vi "SP Determine Active Plot.vi"(0 "CH Index":i32, 1 "Trace Orientation":enum32{"Overlay", "Split"}(radio), 2 "Plot Orientation":enum32{"Single", "Dual", "Quad"}(radio), 3 "Plots Tab Control":refnum<vi>) -> ()   [LabVIEW 2011]
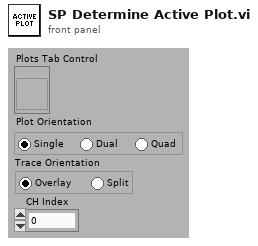
[diagram p1: front panel]
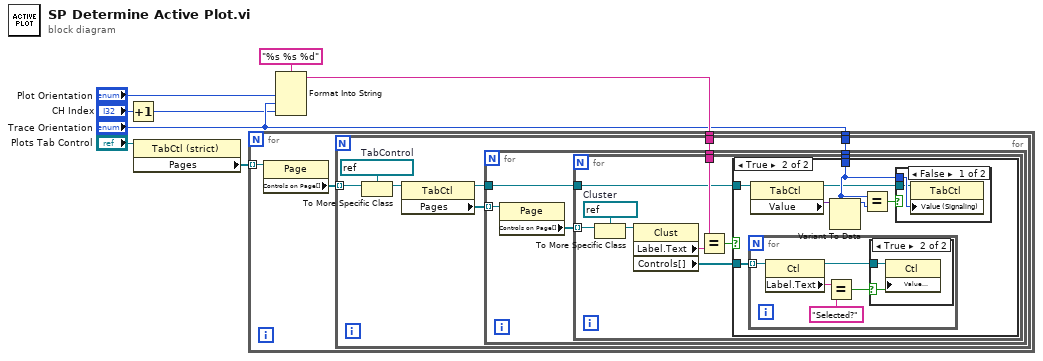
[diagram p0: block diagram]
diagram:
  n1 = Increment(x="CH Index") -> (x+1=w1:i32)
  n2 = property class="TabCtl (strict)"(reference="Plots Tab Control") -> ("Pages"=w4:refnum<vi>[])  [unwired: 1 in, 2 out]
  n3 = Format Into String(format string="%s %s %d", "Plot Orientation", "Trace Orientation", w1) -> (resulting string=w3:string)  [unwired: 2 in, 1 out]
  n4 = for {
    tunnel: w4 -> [w12] mode=indexing
    tunnel: w3 -> [w10]
    tunnel: "Trace Orientation" -> [w9]
    n5 = property class="Page"(reference=w12) -> ("Controls on Page[]"=w11:refnum<vi>[])  [unwired: 1 in, 2 out]
    n6 = for {
      tunnel: w11 -> [w19] mode=indexing
      tunnel: w10 -> [w15]
      tunnel: w9 -> [w13]
      w18 = refnum<vi> refnum  # TabControl
      n7 = To More Specific Class(target class=w18, reference=w19) -> (specific class reference=w17:refnum<vi>)  [unwired: 1 in, 1 out]
      n8 = property class="TabCtl"(reference=w17) -> (reference out=w14:refnum<vi>, "Pages"=w16:refnum<vi>[])  [unwired: 1 in, 1 out]
      n9 = for {
        tunnel: w16 -> [w24] mode=indexing
        tunnel: w15 -> [w22]
        tunnel: w14 -> [w21]
        tunnel: w13 -> [w20]
        n10 = property class="Page"(reference=w24) -> ("Controls on Page[]"=w23:refnum<vi>[])  [unwired: 1 in, 2 out]
        n11 = for {
          tunnel: w23 -> [w32] mode=indexing
          tunnel: w22 -> [w29]
          tunnel: w21 -> [w26]
          tunnel: w20 -> [w25]
          w33 = refnum<vi> refnum  # Cluster
          n12 = To More Specific Class(target class=w33, reference=w32) -> (specific class reference=w31:refnum<vi>)  [unwired: 1 in, 1 out]
          n13 = property class="Clust"(reference=w31) -> ("Label.Text"=w30:string, "Controls[]"=w27:refnum<vi>[])  [unwired: 1 in, 2 out]
          n14 = Equal?(x=w29, y=w30) -> (x = y?=w28:bool)
          n15 = case shown="True" w28 {
            tunnel: w27 -> [_ w40]
            tunnel: w26 -> [_ w39]
            tunnel: w25 -> [_ w37]
            frame False {
            }
            frame True {
              n16 = for {
                tunnel: w40 -> [w47] mode=indexing
                n17 = property class="Ctl"(reference=w47) -> (reference out=w43:refnum<vi>, "Label.Text"=w46:string)  [unwired: 1 in, 1 out]
                n18 = Equal?(x=w46, y="Selected?") -> (x = y?=w44:bool)
                n19 = case shown="True" w44 {
                  selector: w44 -> [_ w48]
                  tunnel: w43 -> [_ w49]
                  frame False {
                  }
                  frame True {
                    n20 = property class="Ctl"(reference=w49, "Value (Signaling)"=w48) -> ()  [unwired: 1 in, 2 out]
                  }
                }
              }
              n21 = property class="TabCtl"(reference=w39) -> (reference out=w34:refnum<vi>, "Value"=w38:variant)  [unwired: 1 in, 1 out]
              n22 = Variant To Data(type=w37, Variant=w38) -> (data=w36:enum32{"Overlay", "Split"})  [unwired: 1 in, 1 out]
              n23 = Equal?(x=w37, y=w36) -> (x = y?=w35:bool)
              n24 = case shown="False" w35 {
                tunnel: w37 -> [w42 _]
                tunnel: w34 -> [w41 _]
                frame False {
                  n25 = property class="TabCtl"(reference=w41, "Value (Signaling)"=w42) -> ()  [unwired: 1 in, 2 out]
                }
                frame True {
                }
              }
            }
          }
        }
      }
    }
  }
